vi "SMTP Email Check File List.vi"(4 "error in (no error)":errorcluster, 7 "attachments":T1(array[cluster])) -> (0 "error out":errorcluster, 3 "attachments out":T1(array[cluster]))   [LabVIEW 2009, in "NewNI_SMTPEmail.lvlib"]
doc: "This VI checks for existence all the files specified in the array of clusters Attachments. Error out cluster has a status value of true in case at least one of the files does not exist."
uses:
  NewNI_SMTPEmail.lvlib
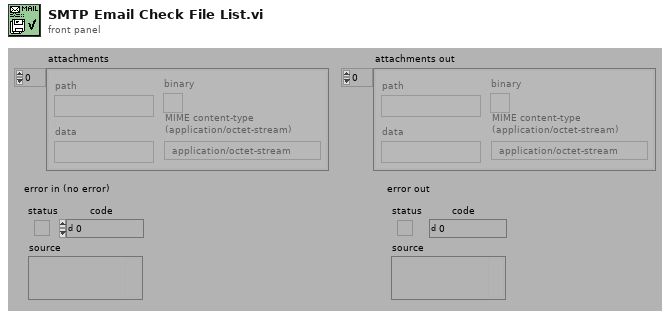
[diagram p1: front panel]
types:
  T1 = cluster{"path":path, "data":string, "binary":bool, "MIME content-type \n(application/octet-stream)":string}[]
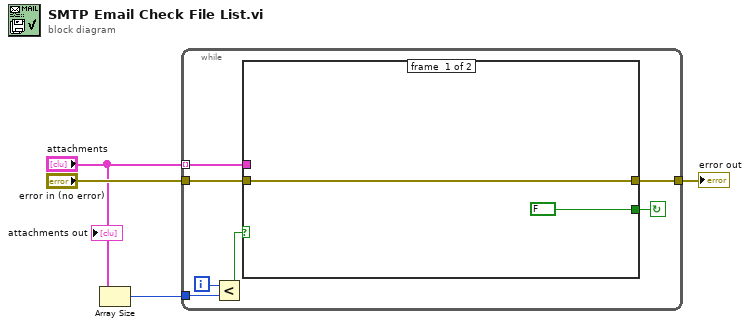
[diagram p0: block diagram]
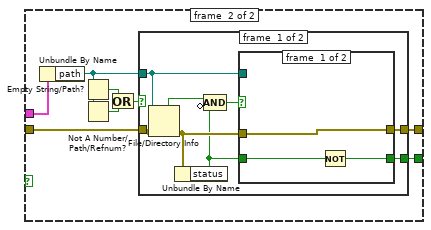
[diagram p2: hidden frame]
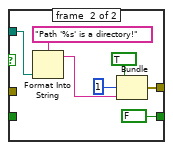
[diagram p3: hidden frame]
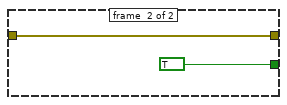
[diagram p4: hidden frame]
diagram:
  n1 = Array Size(array="attachments") -> (size(s)=w3:i32)
  n2 = while {
    tunnel: [w8] -> w2
    tunnel: "error in (no error)" -> [w9]
    tunnel: w3 -> [w10]
    tunnel: "attachments" -> [w7] mode=indexing
    i -> [w11]
    stop <- w5 continue-if-true
    n3 = Less?(x=w11, y=w10) -> (x < y?=w6:bool)
    n4 = case shown="True" w6 {
      tunnel: w7 -> [_ w21]
      tunnel: [w12 w20] -> w8
      tunnel: w9 -> [w12 w19]
      tunnel: [FALSE w18] -> w5
      frame #0 {
      }
      frame #1 {
        n5 = Unbundle By Name(w21) -> ("path"=w15:path)
        n6 = Empty String/Path?(string/path=w15) -> (empty?=w16:bool)
        n7 = Not A Number/Path/Refnum?(number/path/refnum=w15) -> (NaN/Path/Refnum?=w17:bool)
        n8 = Or(x=w16, y=w17) -> (x .or. y?=w14:bool)
        n9 = case shown="False" w14 {
          tunnel: w19 -> [w29 w41]
          tunnel: [w25 w41] -> w20
          tunnel: w15 -> [w22 _]
          tunnel: [w23 TRUE] -> w18
          frame #0 {
            n10 = File/Directory Info(path=w22, error in=w29) -> (directory=w27:bool, error out=w28:errorcluster)  [unwired: 5 out]
            n11 = Unbundle By Name(w28) -> ("status"=w24:bool)
            n12 = Compound Arithmetic op=AND(w27, invert w24) -> (w26:bool)
            n13 = case shown="True" w26 {
              tunnel: w28 -> [w32 _]
              tunnel: [w32 w38] -> w25
              tunnel: w24 -> [w31 _]
              tunnel: [w30 FALSE] -> w23
              tunnel: w22 -> [_ w34]
              frame #0 {
                n14 = Not(x=w31) -> (.not. x?=w30:bool)
              }
              frame #1 {
                n15 = Format Into String(format string="Path '%s' is a directory!", w34) -> (resulting string=w33:string)  [unwired: 2 in, 1 out]
                n16 = Bundle(TRUE, 1, w33) -> (w38:errorcluster)  [unwired: 1 out]
              }
            }
          }
          frame #1 {
          }
        }
      }
    }
  }
  "error out" <- w2
  "attachments out" <- "attachments"
